vi "lone test.vi"   [LabVIEW 2020, in "Unit Tests for Runner.lvclass"]
uses:
  Unit Tests for Runner.lvclass
  classes/Test/Test.lvclass
  classes/Assert/Assert.lvclass
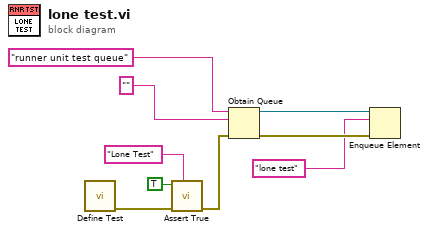
[diagram p0: block diagram]
diagram:
  n1 = call "Define Test.vi"() -> ("error out"=w3:errorcluster)  [unwired: 10 in, 1 out]
  n2 = call "Assert True.vi"("Label"="Lone Test", "error in (no error)"=w3, "True?"=TRUE) -> ("error out"=w2:errorcluster)  [unwired: 7 in, 1 out]
  n3 = Obtain Queue(name (unnamed)="runner unit test queue", element data type="", error in (no error)=w2) -> (queue out=w7:refnum<queue>, error out=w6:errorcluster)  [unwired: 2 in, 1 out]
  n4 = Enqueue Element(queue=w7, element="lone test", error in (no error)=w6) -> ()  [unwired: 1 in, 3 out]
